vi "14 Saving and Reading Files.vi"() -> ()   [LabVIEW 2020]
uses:
  _Subs/OpenDiagram/Open_XControl.xctl
  <vilib>/Utility/file.llb/Write Delimited Spreadsheet (DBL).vi
  <vilib>/Utility/file.llb/Read Delimited Spreadsheet (DBL).vi
panel:
  out "txt files in your temp folder":string[](array[string])
  out "Numbers read":dbl[](array[numeric])
  in  "Numbers to save":dbl[](array[numeric])
  out "Text read":string
  in  "Path to file":path
  in  "OpenDiag":refnum<vi>(xcontrol)
  # "14 Saving and Reading Files\nThis code will save and then read a text file\n\nInstructions:\n1. Select a path (click on the folder icon)\n2. Hit the Run arrow and see the code execute"
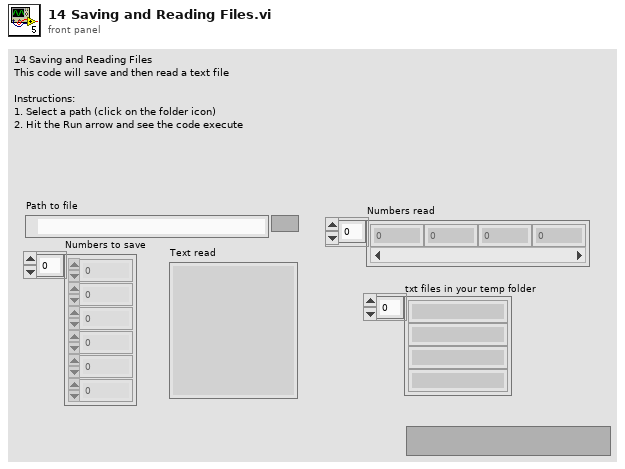
[diagram p1: front panel]
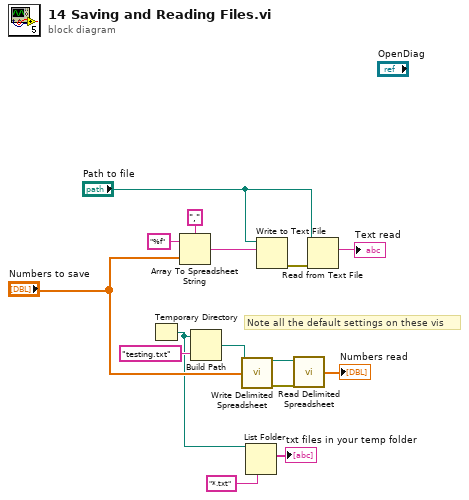
[diagram p0: block diagram]
diagram:
  # "Note all the default settings on these vis"
  n1 = Temporary Directory() -> (w3:path)
  n2 = Array To Spreadsheet String(delimiter (Tab)=",", array="Numbers to save", 3:"%f" ("format string")) -> (spreadsheet string=w10:string)
  n3 = Build Path(base path=w3, name or relative path="testing.txt") -> (appended path=w5:path)
  n4 = call-poly <vilib>:"Write Delimited Spreadsheet.vi"("file path (dialog if empty)"=w5, "1D data"="Numbers to save") -> ("new file path (Not A Path if cancelled)"=w8:path, "error out"=w7:errorcluster)  [unwired: 12 in]
  n5 = List Folder(path=w3, pattern="*.txt") -> (filenames=→"txt files in your temp folder":string[])  [unwired: 2 in, 3 out]
  n6 = Write to Text File(file (use dialog)="Path to file", text=w10) -> (error out=w15:errorcluster)  [unwired: 2 in, 2 out]
  n7 = call-poly <vilib>:"Read Delimited Spreadsheet.vi"("file path (dialog if empty)"=w8, "error in (no error)"=w7) -> ("first row"=→"Numbers read":dbl[])  [unwired: 8 in, 5 out]
  n8 = Read from Text File(file (use dialog)="Path to file", error in=w15) -> (text=→"Text read":string)  [unwired: 2 in, 3 out]
